vi "Create Messages For Registration.vi"(8 "error in (no error)":errorcluster, 10 "Messages MetaData":T1[](array[typedef]), 11 "VI in":refnum<vi>) -> (0 "error out":errorcluster, 3 "VI out":refnum<vi>)   [LabVIEW 2019, in "gRPC Template Creation Utility.lvlib"]
uses:
  gRPC Template Creation Utility.lvlib
  TypeDefs/Message Element Type.ctl
  TypeDefs/Message Element Metadata (Scripting).ctl
  TypeDefs/Message Metadata (Scripting).ctl
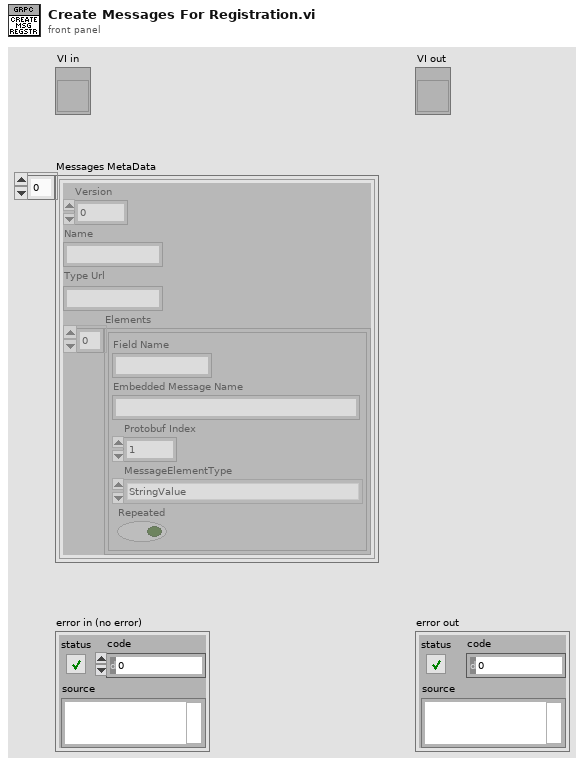
[diagram p1: front panel]
types:
  T1 = typedef "gRPC Template Creation Utility.lvlib/Message Metadata (Scripting).ctl" = cluster{"Version":i32, "Name":string, "Type Url":string, "Elements":T2[]}
  T2 = typedef "gRPC Template Creation Utility.lvlib/Message Element Metadata (Scripting).ctl" = cluster{"Field Name":string, "Embedded Message Name":string, "Protobuf Index":i32, "MessageElementType":T3, "Repeated":bool}
  T3 = typedef "gRPC Template Creation Utility.lvlib/Message Element Type.ctl" = enum32{"Int32Value", "FloatValue", "DoubleValue", "BoolValue", "StringValue", "MessageValue", "Int64Value", "UInt32Value", "UInt64Value", "EnumValue", "Bytes", "Fixed64", "Fixed32", "SFixed64", "SFixed32", "SInt64", "SInt32"}
  T4 = cluster{"Embedded Message Name":string, "Protobuf Index":i32, "MessageElementType":enum32{"Int32Value", "FloatValue", "DoubleValue", "BoolValue", "StringValue", "MessageValue", "Int64Value", "UInt32Value", "UInt64Value", "EnumValue", "Bytes", "Fixed64", "Fixed32", "SFixed64", "SFixed32", "SInt64", "SInt32"}, "Repeated":bool}
  T5 = cluster{"Version":i32, "Name":string, "Type Url":string, "Elements":cluster{"Embedded Message Name":string, "Protobuf Index":i32, "MessageElementType":enum32{"Int32Value", "FloatValue", "DoubleValue", "BoolValue", "StringValue", "MessageValue", "Int64Value", "UInt32Value", "UInt64Value", "EnumValue", "Bytes", "Fixed64", "Fixed32", "SFixed64", "SFixed32", "SInt64", "SInt32"}, "Repeated":bool}[]}
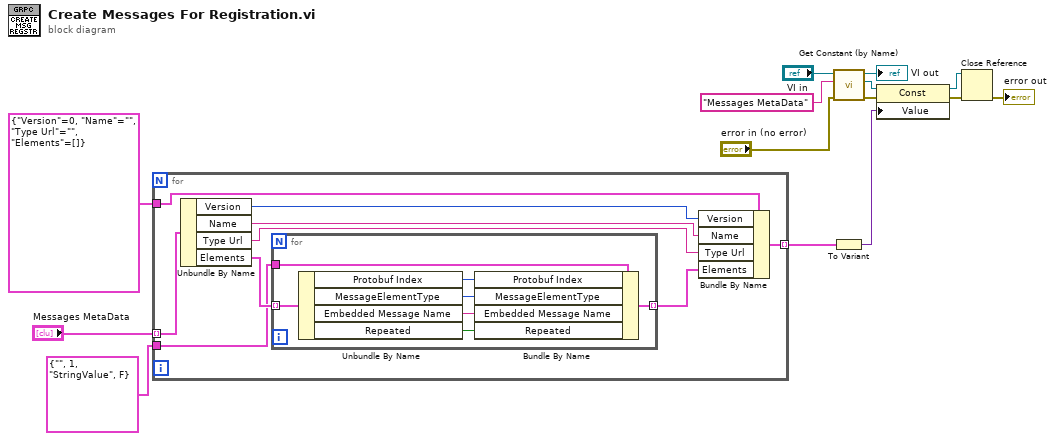
[diagram p0: block diagram]
diagram:
  n1 = for {
    tunnel: "Messages MetaData" -> [w23] mode=indexing
    tunnel: [w21] -> w4 mode=indexing
    tunnel: T4 {"Embedded Message Name"="", "Protobuf Index"=1, "MessageElementType"=enum."StringValue", "Repeated"=FALSE} ("Message Element Metadata") -> [w16]
    tunnel: T5 {"Version"=0, "Name"="", "Type Url"="", "Elements"=[]} ("Message Metadata") -> [w15]
    n2 = Unbundle By Name(w23) -> ("Version"=w17:i32, "Name"=w18:string, "Type Url"=w19:string, "Elements"=w22:T2[])
    n3 = for {
      tunnel: w22 -> [w30] mode=indexing
      tunnel: [w25] -> w20 mode=indexing
      tunnel: w16 -> [w24]
      n4 = Unbundle By Name(w30) -> ("Protobuf Index"=w29:i32, "MessageElementType"=w28:T3, "Embedded Message Name"=w27:string, "Repeated"=w26:bool)
      n5 = Bundle By Name(cluster=w24, "Protobuf Index"=w29, "MessageElementType"=w28, "Embedded Message Name"=w27, "Repeated"=w26) -> (w25:T4)
    }
    n6 = Bundle By Name(cluster=w15, "Version"=w17, "Name"=w18, "Type Url"=w19, "Elements"=w20) -> (w21:T5)
  }
  n7 = call "Get Constant (by Name).vi"("error in (no error)"="error in (no error)", "Constant Label"="Messages MetaData", "Owner VI in"="VI in") -> ("error out"=w9:errorcluster, "Const ref out"=w12:refnum<vi>, "Owner VI out"=→"VI out":refnum<vi>)  [unwired: 5 in, 1 out]
  n8 = To Variant(anything=w4) -> (Variant=w8:variant)
  n9 = property class="Const"(reference=w12, error in=w9, "Value"=w8) -> (reference out=w7:refnum<vi>, error out=w6:errorcluster)
  n10 = Close Reference(reference=w7, error in (no error)=w6) -> (error out=→"error out":errorcluster)
